vi "Untitled 2.vi"() -> ()   [LabVIEW 2015]
uses:
  <vilib>/picture/3D Picture Control/Object/Create Object (name).vi
  <vilib>/picture/3D Picture Control/Object/Add Object (no reference).vi
  <vilib>/picture/3D Picture Control/NI_3D Picture Control.lvlib
panel:
  in  "push":bool
  out "3D Picture":refnum<vi>(3d-picture)
  in  "Translation":cluster{"X":sgl, "Y":sgl, "Z":sgl}
  out "y":dbl
  in  "stop":bool
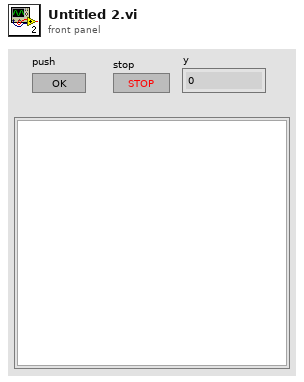
[diagram p1: front panel]
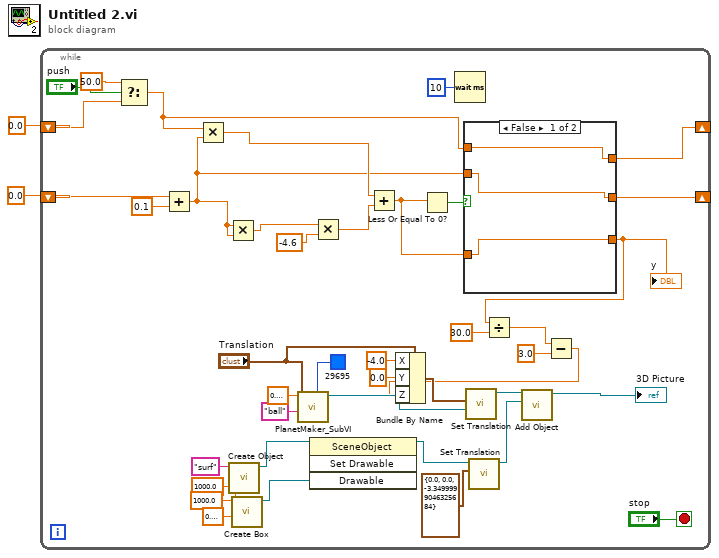
[diagram p0: block diagram]
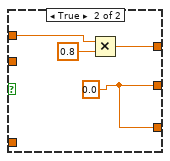
[diagram p2: hidden frame]
diagram:
  n1 = while {
    shift-right: [w36] -> _
    shift-left: 0.0 -> [w4]
    shift-right: [w35] -> _
    shift-left: 0.0 -> [w43]
    stop <- "stop" stop-if-true
    n2 = Select(t=50.0, s="push", f=w4) -> (s? t:f=w3:dbl)
    n3 = Add(x=w43, y=0.1) -> (x+y=w32:dbl)
    n4 = Multiply(x=w3, y=w32) -> (x*y=w38:dbl)
    n5 = Multiply(x=w32, y=w32) -> (x*y=w31:dbl)
    n6 = call-poly <vilib>:"Create Object.vi"("Name"="surf") -> ("Scene:New Object"=w24:refnum<vi>)  [unwired: 9 in, 1 out]
    n7 = call <vilib>:"Create Box.vi"("Length Z"=sgl 0.1, "Length Y"=sgl 1000.0, "Length X"=sgl 1000.0) -> ("New Box Refnum"=w25:refnum<vi>)  [unwired: 7 in, 1 out]
    n8 = call "PlanetMaker_SubVI.vi"("Color"=u32 29695, "Name"="ball", "Translation"="Translation", "Radius"=sgl 0.3) -> ("Rotated Scene Object"=w16:refnum<vi>)  [unwired: 6 in, 1 out]
    n9 = invoke class="SceneObject" method="Set Drawable"(reference=w24, "Drawable"=w25) -> (reference out=w20:refnum<vi>)  [unwired: 2 in, 3 out]
    n10 = Multiply(x=w31, y=-4.6) -> (x*y=w40:dbl)
    n11 = Add(x=w38, y=w40) -> (x+y=w37:dbl)
    n12 = Less Or Equal To 0?(x=w37) -> (x <= 0?=w39:bool)
    n13 = Wait (ms)(milliseconds to wait=u32 10) -> ()  [unwired: 1 out]
    n14 = case shown="False" w39 {
      tunnel: w37 -> [w46 _]
      tunnel: w32 -> [w45 _]
      tunnel: [w44 w49] -> w36
      tunnel: [w45 w48] -> w35
      tunnel: [w46 w48] -> w14
      tunnel: w3 -> [w44 w47]
      frame False {
      }
      frame True {
        w48 = 0.0 ("y")
        n15 = Multiply(x=w47, y=0.8) -> (x*y=w49:dbl)
      }
    }
    "y" <- w14
    n16 = call <vilib>:"Set Translation.vi"("Translation"=cluster{"X":sgl, "Y":sgl, "Z":sgl} {"X"=0.0, "Y"=0.0, "Z"=-3.35}, "Scene Object"=w20) -> ("Translated Object"=w18:refnum<vi>)  [unwired: 8 in, 1 out]
    n17 = Divide(x=w14, y=30.0) -> (x/y=w11:dbl)
    n18 = Subtract(x=w11, y=3.0) -> (x-y=w9:dbl)
    n19 = Bundle By Name(cluster="Translation", "X"=sgl -4.0, "Y"=sgl 0.0, "Z"=w9) -> (w12:cluster{"X":sgl, "Y":sgl, "Z":sgl})
    n20 = call <vilib>:"Set Translation.vi"("Translation"=w12, "Scene Object"=w16) -> ("Translated Object"=w17:refnum<vi>)  [unwired: 8 in, 1 out]
    n21 = call-poly <vilib>:"Add Object.vi"("New Object In"=w18, "Scene Object In"=w17) -> ("Scene Object Out"=→"3D Picture":refnum<vi>)  [unwired: 8 in, 1 out]
  }
